vi "Auto-Refresh Stop.vi"(8 "error in (no error)":errorcluster, 11 "MSX-E3711 in":refnum<class "MSX-E3711.lvclass">) -> (0 "error out":errorcluster, 3 "MSX-E3711 out":refnum<class "MSX-E3711.lvclass">)   [LabVIEW 2014, in "MSX-E3711.lvlib" / "MSX-E3711.lvclass"]
uses:
  MSX-E3711.lvclass
  MSX-E3711.lvclass/MSX-E3711.ctl
  API/MSX-E3711_dll.lvlib
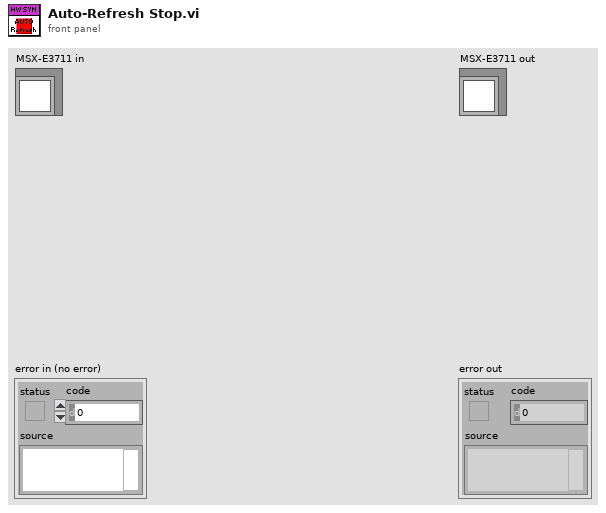
[diagram p1: front panel]
types:
  T1 = typedef "MSX-E3711_dll.lvlib/Connection Data.ctl" = cluster{"MX371x refnum":refnum<k24>, "IP":string, "Connection ID ":refnum<k5>, "MXCommon refnum":refnum<k24>}
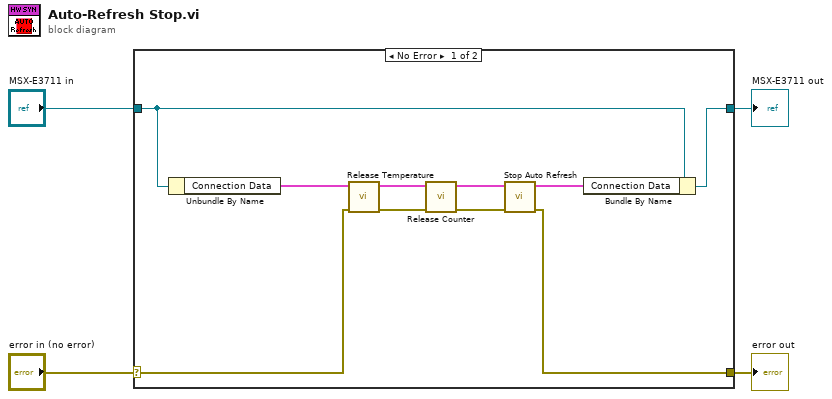
[diagram p0: block diagram]
diagram:
  n1 = case shown="No Error" "error in (no error)" {
    selector: "error in (no error)" -> [w8 w16]
    tunnel: [w5 w16] -> w3
    tunnel: [w13 w15] -> w1
    tunnel: "MSX-E3711 in" -> [w14 w15]
    frame No Error {
      n2 = Unbundle By Name(w14) -> ("Connection Data"=w12:T1)
      n3 = call "Release Temperature.vi"("error in (no error)"=w8, "Connection Data In"=w12) -> ("error out"=w7:errorcluster, "Connection Data Out"=w11:T1)  [unwired: 8 in]
      n4 = call "Release Counter.vi"("error in (no error)"=w7, "Connection Data In"=w11) -> ("error out"=w6:errorcluster, "Connection Data Out"=w10:T1)  [unwired: 8 in]
      n5 = call "Stop Auto Refresh.vi"("error in (no error)"=w6, "Connection Data In"=w10) -> ("error out"=w5:errorcluster, "Connection Data Out"=w9:T1)  [unwired: 8 in]
      n6 = Bundle By Name(cluster=w14, "Connection Data"=w9) -> (w13:refnum<class "MSX-E3711.lvclass">)
    }
    frame Error {
    }
  }
  "error out" <- w3
  "MSX-E3711 out" <- w1
